vi "TCP Test Server.vi"() -> ()   [LabVIEW 2020]
panel:
  in  "IP Address":string="localhost"
  in  "Port":i32=4900
  out "Error":bool
  out "Command":string
  out "Connected":bool
  out "Ready":bool
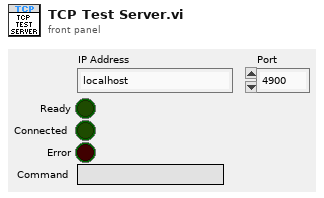
[diagram p1: front panel]
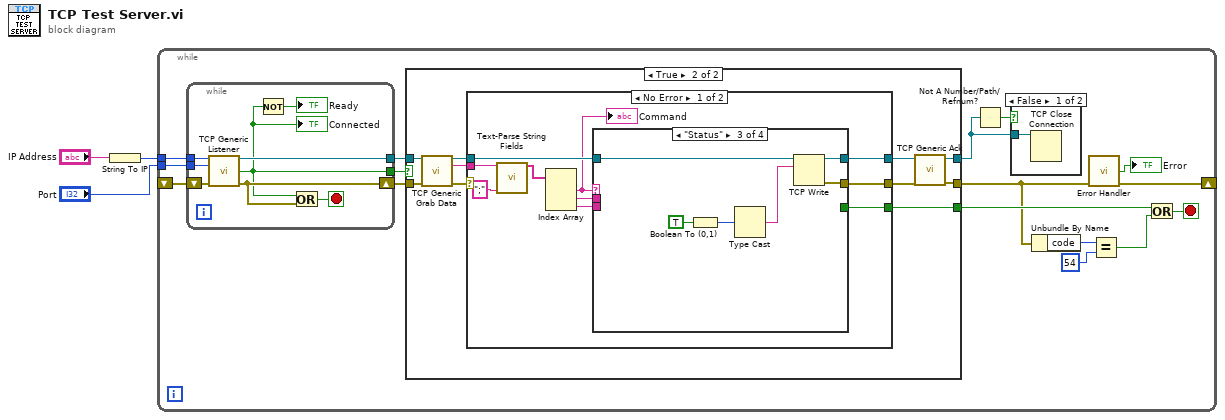
[diagram p0: block diagram]
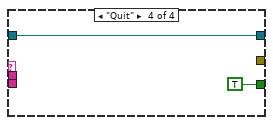
[diagram p6: hidden frame]
diagram:
  n1 = String To IP(1:"IP Address") -> (0:w3:u32)
  n2 = while {
    tunnel: w3 -> [w19]
    tunnel: "Port" -> [w18]
    shift-right: [w8] -> _
    shift-left: _ -> [w17]
    stop <- w5 stop-if-true
    n3 = while {
      tunnel: w19 -> [w62]
      tunnel: w18 -> [w61]
      shift-right: [w58] -> w16
      shift-left: w17 -> [w60]
      tunnel: [w55] -> w15
      tunnel: [w59] -> w14
      stop <- w57 stop-if-true
      n4 = call "TCP Generic Listener.vi"("net address"=w62, "port"=w61, "error in (no error)"=w60) -> ("connection ID"=w59:refnum<k5>, "Connected?"=w55:bool, "error out"=w58:errorcluster)  [unwired: 10 in]
      "Connected" <- w55
      n5 = Not(x=w55) -> (.not. x?=→"Ready":bool)
      n6 = Or(x=w55, y=w58) -> (x .or. y?=w57:bool)
    }
    n7 = case shown="True" w15 {
      tunnel: w16 -> [w21 w31]
      tunnel: w14 -> [w22 w32]
      tunnel: [w22 w25] -> w12
      tunnel: [w21 w24] -> w9
      tunnel: [_ w23] -> w11
      frame False {
      }
      frame True {
        n8 = call "TCP Generic Grab Data.vi"("connection ID"=w32, "error in (no error)"=w31) -> ("connection ID out"=w28:refnum<k5>, "data out"=w30:string, "error out"=w29:errorcluster)  [unwired: 11 in]
        n9 = case shown="No Error" w29 {
          selector: w29 -> [_ w53]
          tunnel: w30 -> [w42 _]
          tunnel: w28 -> [w41 w54]
          tunnel: [w39 w54] -> w27
          tunnel: [w38 w53] -> w26
          tunnel: [w37 _] -> w23
          frame No Error {
            n10 = call "Text-Parse String Fields.vi"("String"=w42, "Separator"=";") -> ("Fields"=w40:string[])  [unwired: 8 in, 5 out]
            n11 = Index Array(array=w40) -> (element #1=w33:string, element #2=w36:string, element #3=w35:string)  [unwired: 3 in]
            "Command" <- w33
            n12 = case shown="\"Status\"" w33 {
              tunnel: w41 -> [w43 w44 w48 w52]
              tunnel: [w43 w44 w50 w52] -> w39
              tunnel: [_ _ w49 _] -> w38
              tunnel: [_ _ _ TRUE] -> w37
              tunnel: w36 -> [_ _ _ _]
              tunnel: w35 -> [_ _ _ _]
              frame "", Default {
              }
              frame "Ping" {
              }
              frame "Status" {
                n13 = Boolean To (0,1)(Boolean=TRUE) -> (0, 1=w46:i16)
                n14 = Type Cast(x=w46) -> (*(type *) &x=w47:string)  [unwired: 1 in]
                n15 = TCP Write(connection ID=w48, data in=w47) -> (connection ID out=w50:refnum<k5>, error out=w49:errorcluster)  [unwired: 2 in, 1 out]
              }
              frame "Quit" {
              }
            }
          }
          frame Error {
          }
        }
        n16 = call "TCP Generic Ack.vi"("connection ID"=w27, "error in (no error)"=w26) -> ("connection ID out"=w25:refnum<k5>, "error out"=w24:errorcluster)  [unwired: 7 in]
      }
    }
    n17 = Not A Number/Path/Refnum?(number/path/refnum=w12) -> (NaN/Path/Refnum?=w13:bool)
    n18 = case shown="False" w13 {
      tunnel: w12 -> [w20 _]
      frame False {
        n19 = TCP Close Connection(connection ID=w20) -> ()  [unwired: 2 in, 2 out]
      }
      frame True {
      }
    }
    n20 = Unbundle By Name(w9) -> ("code"=w7:i32)
    n21 = call "Error Handler.vi"("error in (no error)"=w9) -> ("error?"=→"Error":bool, "No Error"=w8:errorcluster)  [unwired: 12 in, 1 out]
    n22 = Equal?(x=w7, y=54) -> (x = y?=w4:bool)
    n23 = Or(x=w11, y=w4) -> (x .or. y?=w5:bool)
  }
